vi "Load Project.vi"(8 "error in (no error)":errorcluster, 10 "Application in":refnum<data-value>, 11 "DefaltProjectLoader in":refnum<class "ProjectLoader.lvclass">) -> (0 "error out":errorcluster, 1 "Succeed":bool, 2 "Application out":refnum<data-value>, 3 "DefaltProjectLoader out":refnum<class "ProjectLoader.lvclass">)   [LabVIEW 2015, in "ProjectLoader.lvclass"]
uses:
  ProjectLoader.lvclass
  Core/Application.lvclass
  Core/Project.lvclass
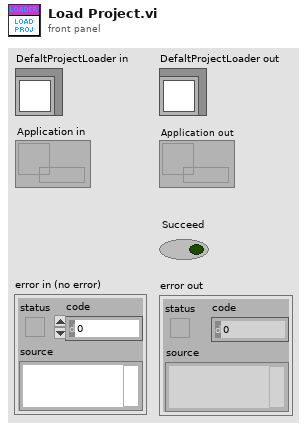
[diagram p1: front panel]
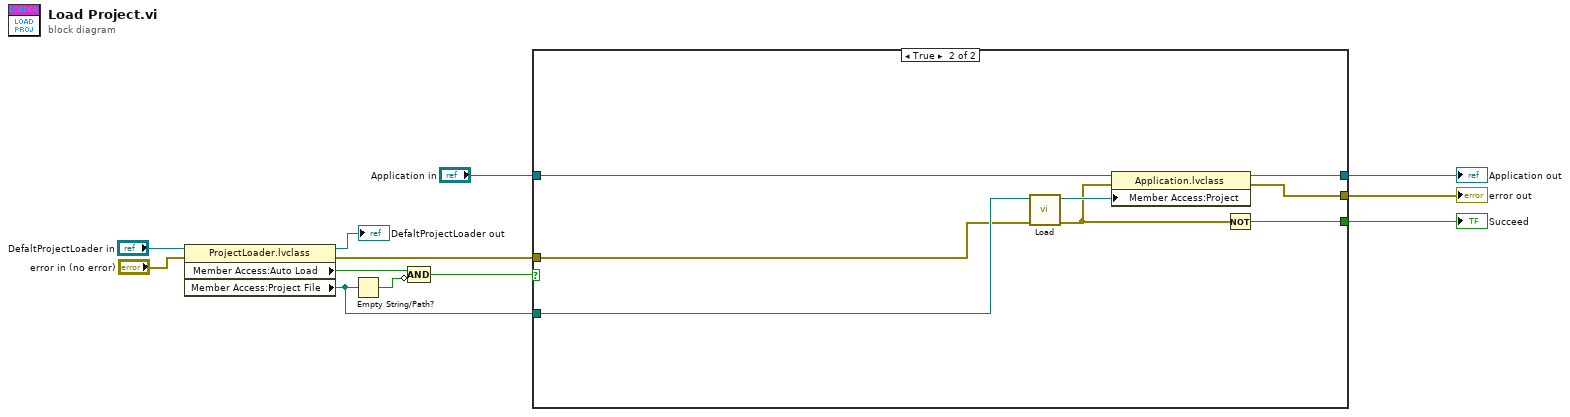
[diagram p0: block diagram]
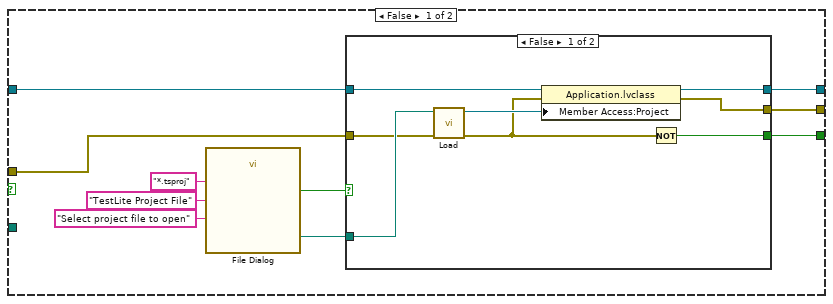
[diagram p2: hidden frame]
diagram:
  n1 = property class="ProjectLoader.lvclass"(reference="DefaltProjectLoader in", error in="error in (no error)") -> (reference out=→"DefaltProjectLoader out":refnum<class "ProjectLoader.lvclass">, error out=w1:errorcluster, "Member Access:Auto Load"=w6:bool, "Member Access:Project File"=w2:path)
  n2 = Empty String/Path?(string/path=w2) -> (empty?=w5:bool)
  n3 = Compound Arithmetic op=AND(w6, invert w5) -> (w3:bool)
  n4 = case shown="True" w3 {
    tunnel: [w22 w33] -> w12
    tunnel: "Application in" -> [w21 w40]
    tunnel: [w20 w39] -> w10
    tunnel: [w14 w34] -> w9
    tunnel: w2 -> [_ w38]
    tunnel: w1 -> [w13 w37]
    frame False {
      n5 = call "File Dialog"("prompt"="Select project file to open", "pattern (all files)"="*.tsproj", "pattern label"="TestLite Project File") -> ("selected path"=w19:path, "cancelled"=w15:bool)  [unwired: 9 in, 2 out]
      n6 = case shown="False" w15 {
        tunnel: w13 -> [w25 w31]
        tunnel: [w30 w31] -> w22
        tunnel: w21 -> [w29 w32]
        tunnel: [w28 w32] -> w20
        tunnel: w19 -> [w27 _]
        tunnel: [w23 _] -> w14
        frame False {
          n7 = call "Load.vi"("error in (no error)"=w25, "Project File"=w27) -> ("error out"=w24:errorcluster, "Project"=w26:refnum<class "Project.lvclass">)  [unwired: 8 in]
          n8 = property class="Application.lvclass"(reference=w29, error in=w24, "Member Access:Project"=w26) -> (reference out=w28:refnum<data-value>, error out=w30:errorcluster)
          n9 = Not(x=w24) -> (.not. x?=w23:bool)
        }
        frame True {
        }
      }
    }
    frame True {
      n10 = call "Load.vi"("error in (no error)"=w37, "Project File"=w38) -> ("error out"=w35:errorcluster, "Project"=w36:refnum<class "Project.lvclass">)  [unwired: 8 in]
      n11 = property class="Application.lvclass"(reference=w40, error in=w35, "Member Access:Project"=w36) -> (reference out=w39:refnum<data-value>, error out=w33:errorcluster)
      n12 = Not(x=w35) -> (.not. x?=w34:bool)
    }
  }
  "error out" <- w12
  "Application out" <- w10
  "Succeed" <- w9
